vi "Get N Pin Information.vi"(8 "error in":errorcluster, 10 "pin or relay names":string[](array[string]), 11 "session reservation":refnum<class "Session Reservation.lvclass">) -> (0 "error out":errorcluster, 1 "pin instruments":refnum<class>[](array[class]), 2 "channel_mappings":T1[](array[typedef]), 3 "session reservation out":refnum<class "Session Reservation.lvclass">)   [LabVIEW 2021, in "Get Pin Information.lvlib"]
uses:
  Get Pin Information.lvlib
  <vilib>/Plug-In SDKs/Clients/Session Management V1/Session Reservation/Session Reservation.lvclass
  <vilib>/gRPC/Generated APIs/ni/measurementlink/sessionmanagement/v1/RPC Messages/ni_measurementlink_sessionmanagement_v1_ChannelMapping.ctl
  <vilib>/Plug-In SDKs/Clients/Session Management V1/Session Reservation/Session Reservation.lvclass/Session Reservation.ctl
  <vilib>/Plug-In SDKs/Clients/Session Management V1/Session Reservation/Get Session Info - NSess .vi
  <vilib>/Plug-In SDKs/Clients/Session Management V1/Session Reservation/Merge Invalid DVR Error.vi
  <vilib>/Plug-In SDKs/Clients/Session Management V1/Session Reservation/Is DVR Valid.vi
  <vilib>/Plug-In SDKs/Measurements/Helpers/Error Strings Global Internal.vi
  <vilib>/Utility/error.llb/Error Cluster From Error Code.vi
  <vilib>/gRPC/Generated APIs/ni/measurementlink/sessionmanagement/v1/ni.measurementlink.sessionmanagement.v1.api.lvlib
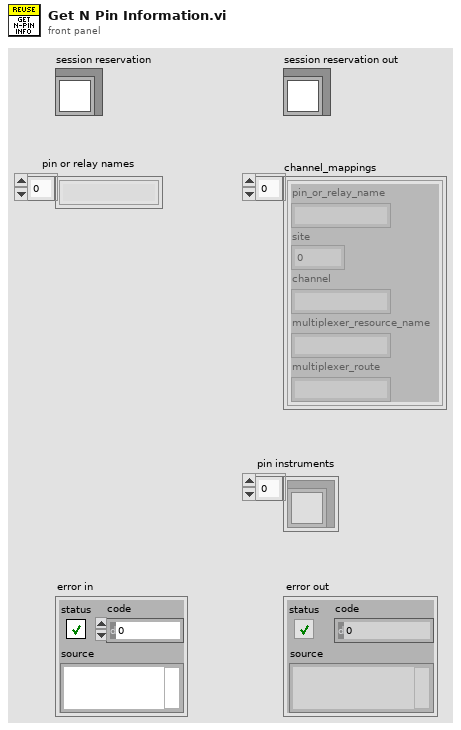
[diagram p1: front panel]
types:
  T1 = typedef "ni.measurementlink.sessionmanagement.v1.api.lvlib/ni_measurementlink_sessionmanagement_v1_ChannelMapping.ctl" = cluster{"pin_or_relay_name":string, "site":i32, "channel":string, "multiplexer_resource_name":string, "multiplexer_route":string}
  T2 = typedef "ni.measurementlink.sessionmanagement.v1.api.lvlib/ni_measurementlink_sessionmanagement_v1_SessionInformation.ctl" = cluster{"session":T3, "resource_name":string, "channel_list":string, "instrument_type_id":string, "session_exists":bool, "channel_mappings":T1[]}
  T3 = typedef "ni.measurementlink.sessionmanagement.v1.api.lvlib/nidevice_grpc_Session.ctl" = cluster{"name":string}
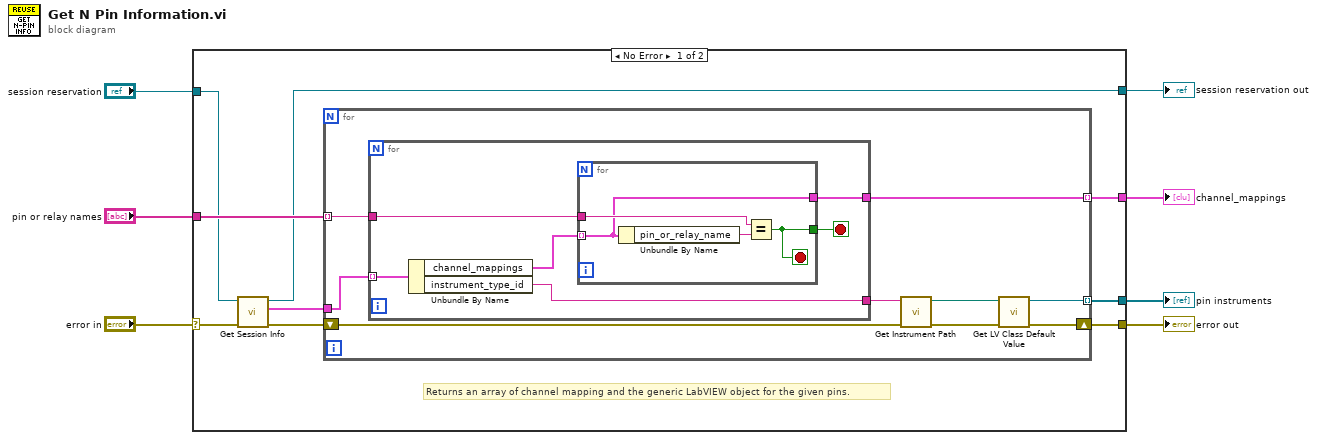
[diagram p0: block diagram]
diagram:
  n1 = case shown="No Error" "error in" {
    selector: "error in" -> [w12 w37]
    tunnel: "pin or relay names" -> [w16 _]
    tunnel: [w15 w37] -> w6
    tunnel: [w14 _] -> w5
    tunnel: "session reservation" -> [w13 w36]
    tunnel: [w9 w36] -> w2
    tunnel: [w8 _] -> w1
    frame No Error {
      # "Returns an array of channel mapping and the generic LabVIEW object for the given pins."
      n2 = call-poly <vilib>:"Get Session Info.vi"("error in"=w12, "session reservation in"=w13) -> ("error out"=w11:errorcluster, "sessions info"=w10:T2[], "session reservation out"=w9:refnum<class "Session Reservation.lvclass">)  [unwired: 7 in]
      n3 = for {
        shift-right: [w22] -> w15
        shift-left: w11 -> [w20]
        tunnel: w16 -> [w24] mode=indexing
        tunnel: w10 -> [w25]
        tunnel: [w23] -> w8 mode=indexing
        tunnel: [w21] -> w14 mode=indexing
        n4 = for {
          tunnel: w25 -> [w31] mode=indexing
          tunnel: [w28] -> w18
          tunnel: [w27] -> w23
          tunnel: w24 -> [w26]
          stop <- w29 stop-if-true
          n5 = Unbundle By Name(w31) -> ("channel_mappings"=w30:T1[], "instrument_type_id"=w28:string)
          n6 = for {
            tunnel: w30 -> [w33] mode=indexing
            tunnel: w26 -> [w35]
            tunnel: [w33] -> w27
            tunnel: [w32] -> w29
            stop <- w32 stop-if-true
            n7 = Unbundle By Name(w33) -> ("pin_or_relay_name"=w34:string)
            n8 = Equal?(x=w35, y=w34) -> (x = y?=w32:bool)
          }
        }
        n9 = call "Get Instrument Path.vi"("error in"=w20, "instrument_type_id"=w18) -> ("error out"=w19:errorcluster, "Instrument Path"=w17:path)  [unwired: 8 in]
        n10 = call <vilib>:"Get LV Class Default Value.vi"("error in (no error)"=w19, "class path"=w17) -> ("error out"=w22:errorcluster, "object"=w21:refnum<class>)  [unwired: 8 in]
      }
    }
    frame Error {
    }
  }
  "error out" <- w6
  "pin instruments" <- w5
  "session reservation out" <- w2
  "channel_mappings" <- w1
